vi "getCategory.vi"(8 "error in (no error)":errorcluster, 11 "Goal in":refnum<class "Goal.lvclass">) -> (0 "error out":errorcluster, 2 "Category.lvclass":refnum<class "Category.lvclass">, 3 "Goal out":refnum<class "Goal.lvclass">)   [LabVIEW 2018, in "Goal.lvclass"]
uses:
  Goal.lvclass
  Category/Category.lvclass
  Goal.lvclass/Goal.ctl
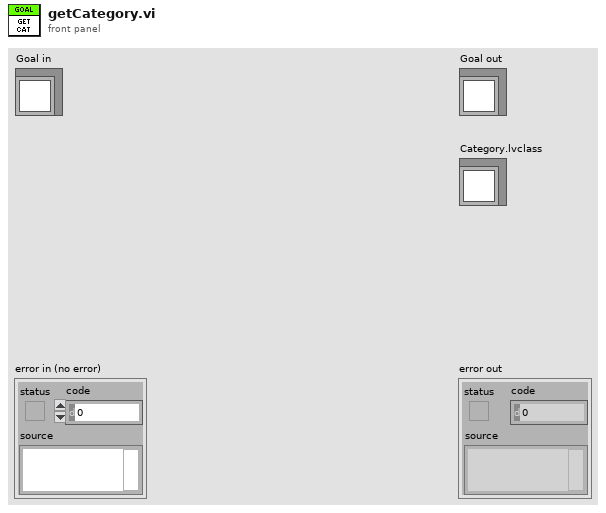
[diagram p1: front panel]
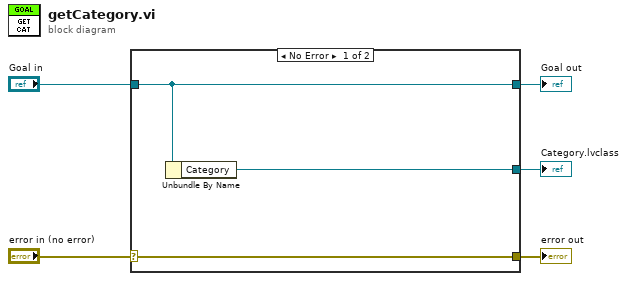
[diagram p0: block diagram]
diagram:
  n1 = case shown="No Error" "error in (no error)" {
    selector: "error in (no error)" -> [w8 w9]
    tunnel: [w8 w9] -> w4
    tunnel: [w7 w10] -> w2
    tunnel: "Goal in" -> [w7 w10]
    tunnel: [w6 _] -> w1
    frame No Error {
      n2 = Unbundle By Name(w7) -> ("Category"=w6:refnum<class "Category.lvclass">)
    }
    frame Error {
    }
  }
  "error out" <- w4
  "Goal out" <- w2
  "Category.lvclass" <- w1
